vi "Remove Bad Scans Spectra.vi"(8 "Bad Scan":bool, 10 "Spectral Data In":T2={"PDT Amp [v]"=0.0, "RIS Amp [v]"=0.0, "B-Field"=[], "All In-Phase Scan Spectra"=[], "Model Select"=enum."OneCompRISTwoPDT", "Fit Each Scan"=FALSE, "PDT Center [g]"=0.0, "In-Phase Average Spectra"=[], "In-Phase Median Spectra"=[], "Out-Phase Median Spectra"=[], "Out-Phase Average Spectra"=[], "Fit Spectra"=[], "Fit No-Baseline Spectra"=[], "All Out-Phase Scan Spectra"=[], "Baseline Offset Correction"=FALSE, "In-Phase Offset [v]"=0.0, "Out-Phase Offset [v]"=0.0, "Ch2 Input\n(Balance)"=[], "Ch3 Input\n(Phase)"=[], "Ch4 Input\n(AFC)"=[], "Fit Pars"=[], "Fit Pars Errors"=[], "Fit Pars Labels"=[], "Raw Scan DAQ Data"=[], "Bad Scans Indicies"=[], "Good In-Phase Scan Spectra"=[], "Good Out-Phase Scan Spectra"=[], "Bad In-Phase Scan Spectra"=[], "Bad Out-Phase Scan Spectra"=[], "Number of bad scans"=0, "Fit History"=[], "PDT Amp. History/Set [v]"=[], "RIS Amp. History/Set [v]"=[], "RIS Amp. History/Scan [v]"=[], "All Shifted B-Fields"=[], "Good Shifted B-Fields"=[], "Ch5 Input\n(SpO2)"=[], "Ch6 Input\n(BPM)"=[], "Global SNR"=0.0, "Fit Error History"=[], "SNR History"=[]} {"Global SNR" min=0.0; "PDT Center [g]" min=0.0; "RIS Amp [v]" min=0.0}, 11 "Acquisition Parameters":T1={"Magnet Angle [deg]"=0.0, "Magnet Angles [deg]"=[], "DeltaVpp [v]"=0.0, "SEM [v]"=0.0, "DeltaVpp Thresh [v]"=0.0, "SEM Thresh [v]"=0.0, "Adaptive Processing"=FALSE, "Acquire Q"=FALSE, "Acquire Photos"=FALSE, "Adaptive Tuning"=FALSE, "Automated Matching"=FALSE, "X-Gradient [G/mm]"=0.0, "Y-Gradient [G/mm]"=0.0, "Z-Gradient [G/mm]"=0.0, "Central Field [G]"=0.0, "Scan Width [G]"=0.0, "Mod. Amp. [G]"=0.0, "Scan Time [s]"=0.0, "Pre-Scan Delay [ms]"=0, "Measurement Timeout [s]"=0.0, "Electromagnet Main Field [G]"=0.0, "Locked Central Field [G]"=0.0, "Scans Excluded"=0, "Scans Completed"=0, "No. Scans/Set"=0, "No. Scans for SNR"=0, "Field Locked Frequency [GHz]"=0.0, "Auto Set-based Field Center"=FALSE, "Prompt for oxy acquisition updates"=FALSE, "Oxy QA Scan?"=FALSE, "Exclude Bad Data"=FALSE, "Optimizing RF Power"=FALSE, "Gradients on/off"=TRUE, "Running Script"=FALSE, "Opto-Coupler Current [A]"=0.0, "Continuous Sweeping"=FALSE, "Sweep Rise Time [sec]"=0, "Reverse Sweep Central Field [G]"=0.0, "Forward Sweep Central Field [G]"=0.0, "Sweep Calibrated"=FALSE, "Modulation Calibrated"=FALSE, "First CheckCal Scan?"=FALSE, "AFC Field Correction"=FALSE, "OxyQAInit Scan Width [G]"=0.0, "OxyQAInit Mod. Amp. [G]"=0.0, "Scans Completed/Session"=0, "Acquire SpO2"=FALSE, "Acquire Temperature"=FALSE, "Over Mod"=FALSE} {"OxyQAInit Mod. Amp. [G]" min=0.0; "OxyQAInit Scan Width [G]" min=0.0; "Mod. Amp. [G]" min=0.0; "Scan Width [G]" min=0.0; "Measurement Timeout [s]" min=0.0; "Scan Time [s]" min=0.0; "Z-Gradient [G/mm]" min=0.0; "Y-Gradient [G/mm]" min=0.0; "X-Gradient [G/mm]" min=0.0; "SEM Thresh [v]" min=0.0; "DeltaVpp Thresh [v]" min=0.0; "SEM [v]" min=0.0}) -> (2 "Spectral Data Out":T2={"PDT Amp [v]"=0.0, "RIS Amp [v]"=0.0, "B-Field"=[], "All In-Phase Scan Spectra"=[], "Model Select"=enum."OneCompRISTwoPDT", "Fit Each Scan"=FALSE, "PDT Center [g]"=0.0, "In-Phase Average Spectra"=[], "In-Phase Median Spectra"=[], "Out-Phase Median Spectra"=[], "Out-Phase Average Spectra"=[], "Fit Spectra"=[], "Fit No-Baseline Spectra"=[], "All Out-Phase Scan Spectra"=[], "Baseline Offset Correction"=FALSE, "In-Phase Offset [v]"=0.0, "Out-Phase Offset [v]"=0.0, "Ch2 Input\n(Balance)"=[], "Ch3 Input\n(Phase)"=[], "Ch4 Input\n(AFC)"=[], "Fit Pars"=[], "Fit Pars Errors"=[], "Fit Pars Labels"=[], "Raw Scan DAQ Data"=[], "Bad Scans Indicies"=[], "Good In-Phase Scan Spectra"=[], "Good Out-Phase Scan Spectra"=[], "Bad In-Phase Scan Spectra"=[], "Bad Out-Phase Scan Spectra"=[], "Number of bad scans"=0, "Fit History"=[], "PDT Amp. History/Set [v]"=[], "RIS Amp. History/Set [v]"=[], "RIS Amp. History/Scan [v]"=[], "All Shifted B-Fields"=[], "Good Shifted B-Fields"=[], "Ch5 Input\n(SpO2)"=[], "Ch6 Input\n(BPM)"=[], "Global SNR"=0.0, "Fit Error History"=[], "SNR History"=[]} {"Global SNR" min=0.0; "PDT Center [g]" min=0.0; "RIS Amp [v]" min=0.0})   [LabVIEW 2016]
uses:
  Types/Spectral Data.ctl
  Types/Fitting Model Selection.ctl
  Types/Acquisition Parameters.ctl
panel:
  # "Gradients"
  # "Field"
  # "Scans and Sets"
  # "Timing"
  # "Adaptive Dosimetric \nData Processing"
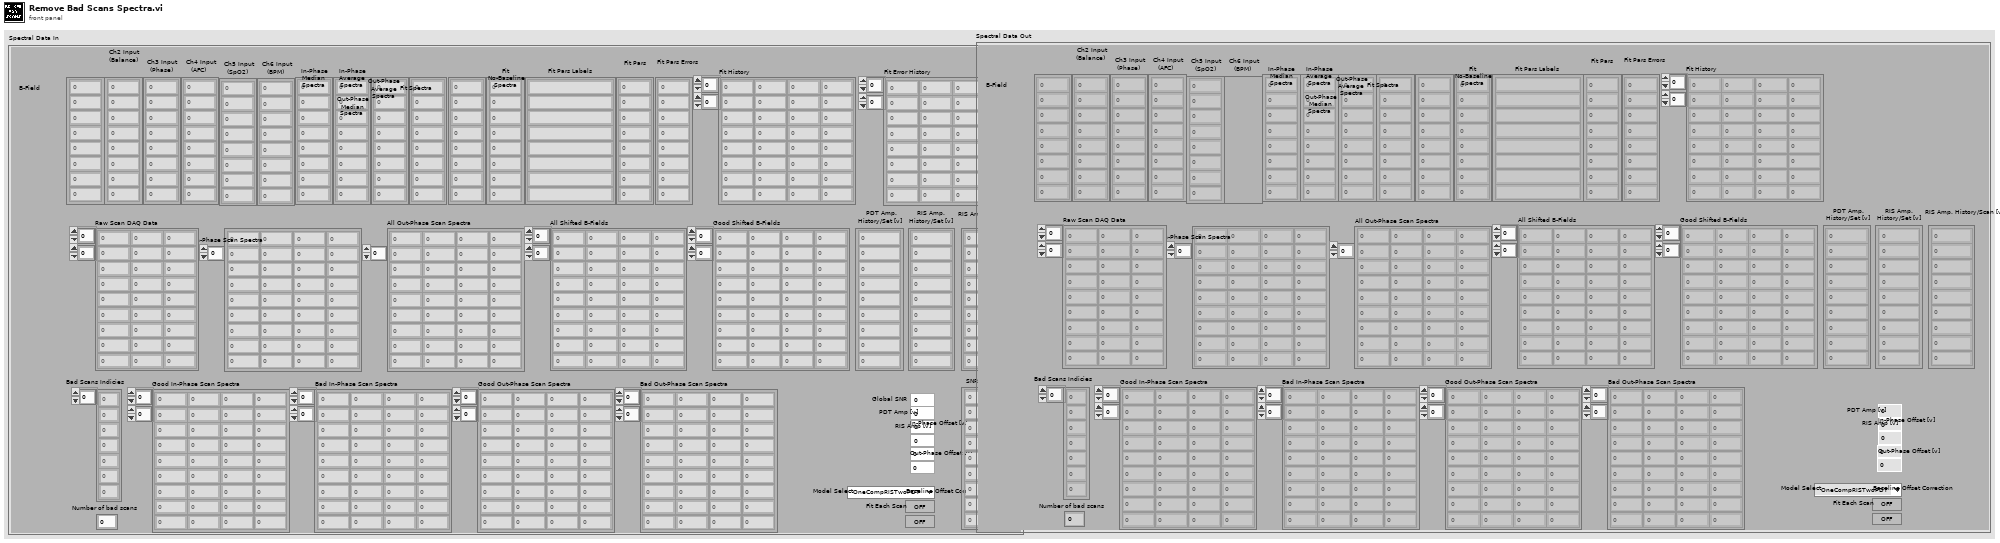
[diagram p1: front panel]
types:
  T1 = typedef "Acquisition Parameters.ctl" = cluster{"Magnet Angle [deg]":dbl, "Magnet Angles [deg]":dbl[], "DeltaVpp [v]":dbl, "SEM [v]":dbl, "DeltaVpp Thresh [v]":dbl, "SEM Thresh [v]":dbl, "Adaptive Processing":bool, "Acquire Q":bool, "Acquire Photos":bool, "Adaptive Tuning":bool, "Automated Matching":bool, "X-Gradient [G/mm]":dbl, "Y-Gradient [G/mm]":dbl, "Z-Gradient [G/mm]":dbl, "Central Field [G]":dbl, "Scan Width [G]":dbl, "Mod. Amp. [G]":dbl, "Scan Time [s]":dbl, "Pre-Scan Delay [ms]":u32, "Measurement Timeout [s]":dbl, "Electromagnet Main Field [G]":dbl, "Locked Central Field [G]":dbl, "Scans Excluded":u32, "Scans Completed":u32, "No. Scans/Set":u32, "No. Scans for SNR":u32, "Field Locked Frequency [GHz]":dbl, "Auto Set-based Field Center":bool, "Prompt for oxy acquisition updates":bool, "Oxy QA Scan?":bool, "Exclude Bad Data":bool, "Optimizing RF Power":bool, "Gradients on/off":bool, "Running Script":bool, "Opto-Coupler Current [A]":dbl, "Continuous Sweeping":bool, "Sweep Rise Time [sec]":u32, "Reverse Sweep Central Field [G]":dbl, "Forward Sweep Central Field [G]":dbl, "Sweep Calibrated":bool, "Modulation Calibrated":bool, "First CheckCal Scan?":bool, "AFC Field Correction":bool, "OxyQAInit Scan Width [G]":dbl, "OxyQAInit Mod. Amp. [G]":dbl, "Scans Completed/Session":u32, "Acquire SpO2":bool, "Acquire Temperature":bool, "Over Mod":bool}
  T2 = typedef "Spectral Data.ctl" = cluster{"PDT Amp [v]":dbl, "RIS Amp [v]":dbl, "B-Field":dbl[], "All In-Phase Scan Spectra":dbl[][], "Model Select":T3, "Fit Each Scan":bool, "PDT Center [g]":dbl, "In-Phase Average Spectra":dbl[], "In-Phase Median Spectra":dbl[], "Out-Phase Median Spectra":dbl[], "Out-Phase Average Spectra":dbl[], "Fit Spectra":dbl[], "Fit No-Baseline Spectra":dbl[], "All Out-Phase Scan Spectra":dbl[][], "Baseline Offset Correction":bool, "In-Phase Offset [v]":dbl, "Out-Phase Offset [v]":dbl, "Ch2 Input\n(Balance)":dbl[], "Ch3 Input\n(Phase)":dbl[], "Ch4 Input\n(AFC)":dbl[], "Fit Pars":dbl[], "Fit Pars Errors":dbl[], "Fit Pars Labels":string[], "Raw Scan DAQ Data":dbl[][], "Bad Scans Indicies":i32[], "Good In-Phase Scan Spectra":dbl[][], "Good Out-Phase Scan Spectra":dbl[][], "Bad In-Phase Scan Spectra":dbl[][], "Bad Out-Phase Scan Spectra":dbl[][], "Number of bad scans":i32, "Fit History":dbl[][], "PDT Amp. History/Set [v]":dbl[], "RIS Amp. History/Set [v]":dbl[], "RIS Amp. History/Scan [v]":dbl[], "All Shifted B-Fields":dbl[][], "Good Shifted B-Fields":dbl[][], "Ch5 Input\n(SpO2)":dbl[], "Ch6 Input\n(BPM)":dbl[], "Global SNR":dbl, "Fit Error History":dbl[][], "SNR History":dbl[]}
  T3 = typedef "Fitting Model Selection.ctl" = enum16{"OneCompRIS", "OneCompRISTwoPDT", "OneCompRISRev", "OneCompRISTwoPDTRev", "LiPc", "TwoLiPc", "ThreeLiPc", "FourLiPc", "PDTCalibration", "CE_Ink", "Printex", "MelaninTwoPDT"}
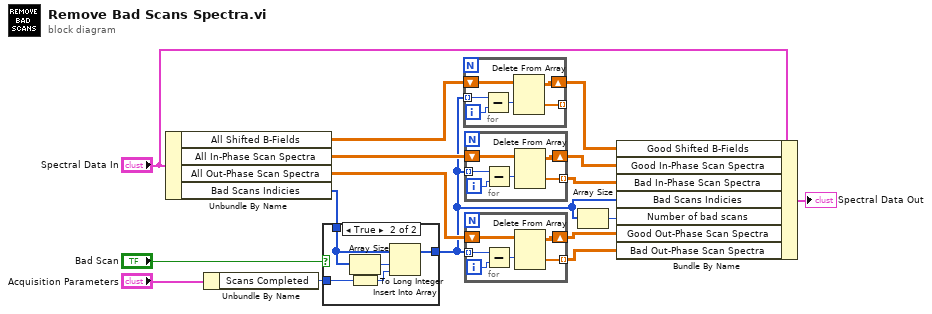
[diagram p0: block diagram]
diagram:
  n1 = Unbundle By Name("Spectral Data In") -> ("All Shifted B-Fields"=w6:dbl[][], "All In-Phase Scan Spectra"=w15:dbl[][], "All Out-Phase Scan Spectra"=w16:dbl[][], "Bad Scans Indicies"=w8:i32[])
  n2 = Unbundle By Name("Acquisition Parameters") -> ("Scans Completed"=w2:u32)
  n3 = case shown="True" "Bad Scan" {
    tunnel: w8 -> [w17 w21]
    tunnel: [w17 w20] -> w5
    tunnel: w2 -> [_ w19]
    frame False {
    }
    frame True {
      n4 = Array Size(array=w21) -> (size(s)=w22:i32)
      n5 = To Long Integer(number=w19) -> (32bit integer=w18:i32)
      n6 = Insert Into Array(array=w21, index=w22, new element=w18) -> (w20:i32[])
    }
  }
  n7 = for {
    shift-right: [w27] -> w4
    shift-left: w6 -> [w28]
    tunnel: [w26] -> _ mode=indexing
    tunnel: w5 -> [w25] mode=indexing
    i -> [w23]
    n8 = Subtract(x=w25, y=w23) -> (x-y=w24:i32)
    n9 = Delete From Array(array=w28, index (row)=w24) -> (deleted portion=w26:dbl[], array with subset deleted=w27:dbl[][])  [unwired: 2 in]
  }
  n10 = for {
    shift-right: [w33] -> w14
    shift-left: w15 -> [w34]
    tunnel: [w32] -> w13 mode=indexing
    tunnel: w5 -> [w31] mode=indexing
    i -> [w29]
    n11 = Subtract(x=w31, y=w29) -> (x-y=w30:i32)
    n12 = Delete From Array(array=w34, index (row)=w30) -> (deleted portion=w32:dbl[], array with subset deleted=w33:dbl[][])  [unwired: 2 in]
  }
  n13 = for {
    shift-right: [w39] -> w12
    shift-left: w16 -> [w40]
    tunnel: [w38] -> w11 mode=indexing
    tunnel: w5 -> [w37] mode=indexing
    i -> [w35]
    n14 = Subtract(x=w37, y=w35) -> (x-y=w36:i32)
    n15 = Delete From Array(array=w40, index (row)=w36) -> (deleted portion=w38:dbl[], array with subset deleted=w39:dbl[][])  [unwired: 2 in]
  }
  n16 = Array Size(array=w5) -> (size(s)=w7:i32)
  n17 = Bundle By Name(cluster="Spectral Data In", "Good Shifted B-Fields"=w4, "Good In-Phase Scan Spectra"=w14, "Bad In-Phase Scan Spectra"=w13, "Bad Scans Indicies"=w5, "Number of bad scans"=w7, "Good Out-Phase Scan Spectra"=w12, "Bad Out-Phase Scan Spectra"=w11) -> (→"Spectral Data Out":T2)
